vi "Event Handle Loop_Draw_Close Button.vi"(8 "error in (no error)":errorcluster, 10 "Picture In":picture, 11 "QMenu Class in":refnum<class "QMenu Class.lvclass">) -> (0 "error out":errorcluster, 2 "Picture Out":picture, 3 "QMenu Class out":refnum<class "QMenu Class.lvclass">)   [LabVIEW 2020, in "QTab.lvlib" / "QMenu Class.lvclass"]
uses:
  QMenu Class.lvclass
  QMenu Class.lvclass/QMenu Class.ctl
  Read Close Button Image.vi
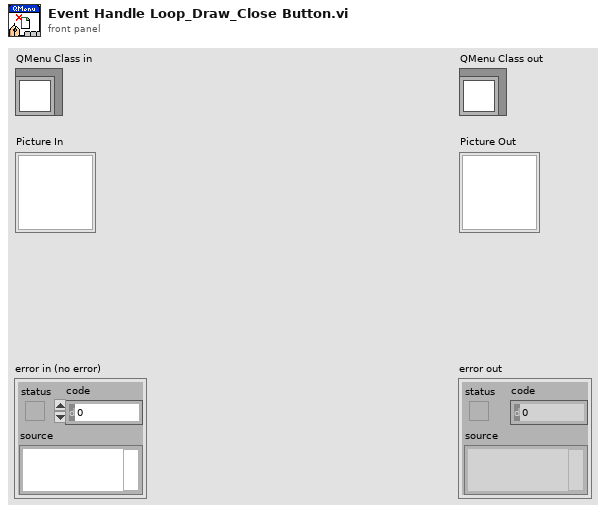
[diagram p1: front panel]
types:
  T1 = typedef "imagedata.ctl" = cluster{"image type":i32, "image depth":i32, "image":u8[], "mask":u8[], "colors":u32[], "Rectangle":cluster{"left":i16, "top":i16, "right":i16, "bottom":i16}}
  T2 = cluster{"left":i16, "top":i16, "right":i16, "bottom":i16}
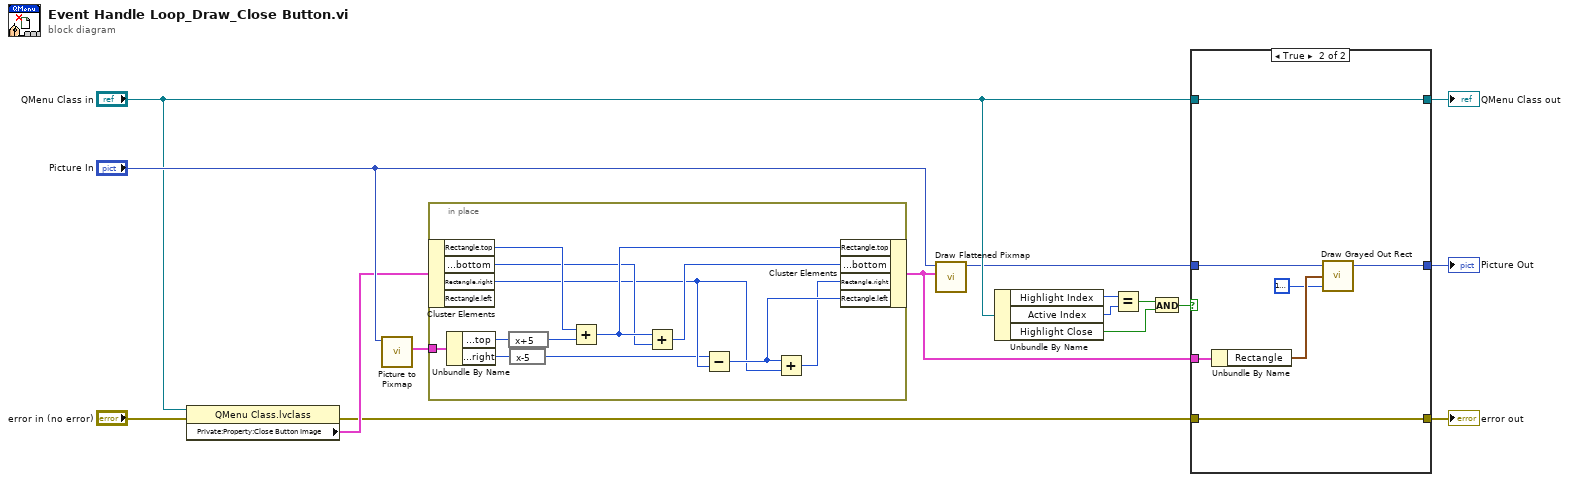
[diagram p0: block diagram]
diagram:
  n1 = property class="QMenu Class.lvclass"(reference="QMenu Class in", error in="error in (no error)") -> (error out=w12:errorcluster, "Private:Property:Close Button Image"=w13:T1)  [unwired: 1 out]
  n2 = call <vilib>:"Picture to Pixmap.vi"("picture"="Picture In") -> ("image data"=w14:T1)  [unwired: 9 in, 1 out]
  n3 = in-place {
    in-place-border: w14 -> [w28]
    n4 = in-place-cluster #1(w13) -> ("Rectangle.top"=w27:i16, "Rectangle.bottom"=w23:i16, "Rectangle.right"=w19:i16)  [unwired: 1 out]
    n5 = Unbundle By Name(w28) -> ("Rectangle.top"=w26:i16, "Rectangle.right"=w18:i16)
    n6 = expression code="x+5"(w26) -> (w25:i16)
    n7 = expression code="x-5"(w18) -> (w17:i16)
    n8 = Add(x=w27, y=w25) -> (x+y=w24:i16)
    n9 = Add(x=w24, y=w23) -> (x+y=w22:i16)
    n10 = Subtract(x=w17, y=w19) -> (x-y=w21:i16)
    n11 = Add(x=w21, y=w19) -> (x+y=w20:i16)
    n12 = in-place-cluster #1("Rectangle.top"=w24, "Rectangle.bottom"=w22, "Rectangle.right"=w20, "Rectangle.left"=w21) -> (w7:T1)
  }
  n13 = call <vilib>:"Draw Flattened Pixmap.vi"("image data"=w7, "picture"="Picture In") -> ("new picture"=w8:picture)  [unwired: 7 in]
  n14 = Unbundle By Name("QMenu Class in") -> ("Highlight Index"=w5:i32, "Active Index"=w4:i32, "Highlight Close"=w2:bool)
  n15 = Equal?(x=w5, y=w4) -> (x = y?=w3:bool)
  n16 = And(x=w3, y=w2) -> (x .and. y?=w1:bool)
  n17 = case shown="True" w1 {
    tunnel: w12 -> [w30 w38]
    tunnel: [w30 w38] -> w11
    tunnel: "QMenu Class in" -> [w29 w37]
    tunnel: [w29 w37] -> w9
    tunnel: w8 -> [w31 w35]
    tunnel: w7 -> [_ w36]
    tunnel: [w31 w32] -> w6
    frame False {
    }
    frame True {
      n18 = Unbundle By Name(w36) -> ("Rectangle"=w34:T2)
      n19 = call <vilib>:"Draw Grayed Out Rect.vi"("color(black)"=u32 16777225, "rect"=w34, "picture"=w35) -> ("new picture"=w32:picture)  [unwired: 2 in]
    }
  }
  "error out" <- w11
  "QMenu Class out" <- w9
  "Picture Out" <- w6
